vi "Unregister Next Button Visibility.vi"(8 "error in (no error)":errorcluster, 10 "View Enqueuer":refnum<class "Message Enqueuer.lvclass">, 11 "Project Model in":refnum<class "Project Model.lvclass">) -> (0 "error out":errorcluster, 3 "Project Model out":refnum<class "Project Model.lvclass">)   [LabVIEW 2013, in "Project Model.lvlib" / "Project Model.lvclass"]
uses:
  Project Model.lvclass
  <vilib>/ActorFramework/Message Enqueuer/Message Enqueuer.lvclass
  Project Model.lvclass/Project Model.ctl
  <vilib>/ActorFrameworkMVC/View Observer/View Registry/View Registry.lvclass
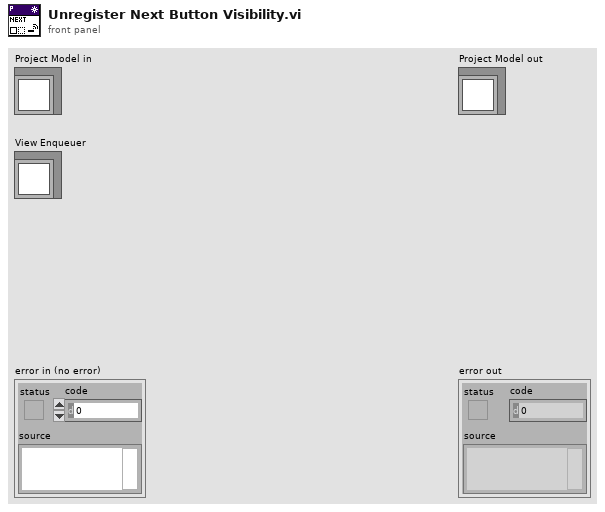
[diagram p1: front panel]
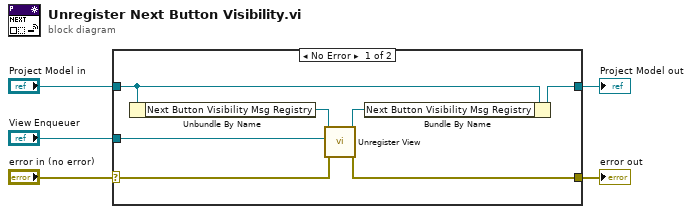
[diagram p0: block diagram]
diagram:
  n1 = case shown="No Error" "error in (no error)" {
    selector: "error in (no error)" -> [w9 w14]
    tunnel: "Project Model in" -> [w12 w13]
    tunnel: "View Enqueuer" -> [w11 _]
    tunnel: [w10 w13] -> w2
    tunnel: [w6 w14] -> w1
    frame No Error {
      n2 = Unbundle By Name(w12) -> ("Next Button Visibility Msg Registry"=w8:refnum<class "View Registry.lvclass">)
      n3 = call <vilib>:"Unregister View.vi"("error in (no error)"=w9, "View Enqueuer"=w11, "View Registry in"=w8) -> ("error out"=w6:errorcluster, "View Registry out"=w7:refnum<class "View Registry.lvclass">)  [unwired: 7 in]
      n4 = Bundle By Name(cluster=w12, "Next Button Visibility Msg Registry"=w7) -> (w10:refnum<class "Project Model.lvclass">)
    }
    frame Error {
    }
  }
  "error out" <- w1
  "Project Model out" <- w2
